vi "Write Notifier.vi"(8 "error in (no error)":errorcluster, 10 "notifier":refnum<notifier>, 11 "Basic Test Manager in":refnum<class "Basic Test Manager.lvclass">) -> (0 "error out":errorcluster, 3 "Basic Test Manager out":refnum<class "Basic Test Manager.lvclass">)   [LabVIEW 2013, in "Caraya.lvlib" / "Basic Test Manager.lvclass"]
uses:
  Basic Test Manager.lvclass
  subVIs/Test Notification.ctl
  Basic Test Manager.lvclass/Basic Test Manager.ctl
  Caraya.lvlib
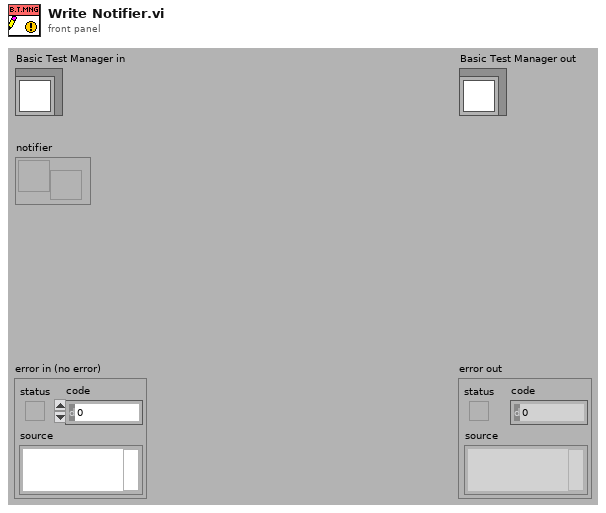
[diagram p1: front panel]
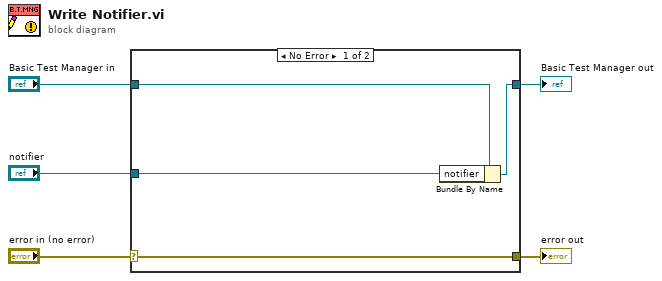
[diagram p0: block diagram]
diagram:
  n1 = case shown="No Error" "error in (no error)" {
    selector: "error in (no error)" -> [w9 w10]
    tunnel: [w9 w10] -> w4
    tunnel: [w7 w11] -> w2
    tunnel: "Basic Test Manager in" -> [w8 w11]
    tunnel: "notifier" -> [w6 _]
    frame No Error {
      n2 = Bundle By Name(cluster=w8, "notifier"=w6) -> (w7:refnum<class "Basic Test Manager.lvclass">)
    }
    frame Error {
    }
  }
  "error out" <- w4
  "Basic Test Manager out" <- w2
